vi "InitProgressLauncher.vi"(7 "InitProgRef":refnum<vi>, 13 "EscapeRef":refnum<vi>) -> ()   [LabVIEW 2019]
panel:
  out "error out":errorcluster
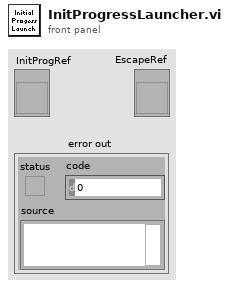
[diagram p1: front panel]
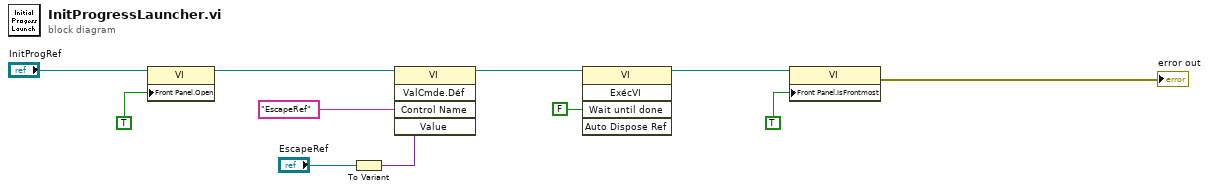
[diagram p0: block diagram]
diagram:
  n1 = property class="VI"(reference="InitProgRef", "Front Panel.Open"=TRUE ("Front Panel Window:Open")) -> (reference out=w2:refnum<vi>)  [unwired: 1 in, 1 out]
  n2 = To Variant(anything="EscapeRef") -> (Variant=w9:variant)
  n3 = invoke class="VI" method="ValCmde.Déf"(reference=w2, "Control Name"="EscapeRef" ("Name"), "Value"=w9) -> (reference out=w5:refnum<vi>)  [unwired: 2 in, 4 out]
  n4 = invoke class="VI" method="ExécVI"(reference=w5, "Wait until done"=FALSE ("Wait Until Done")) -> (reference out=w1:refnum<vi>)  [unwired: 3 in, 4 out]
  n5 = property class="VI"(reference=w1, "Front Panel.IsFrontmost"=TRUE ("Front Panel Window:Is Frontmost")) -> (error out=→"error out":errorcluster)  [unwired: 1 in, 1 out]
